vi "TAT_LABVIEW_TO_PLC_St2.vi"(7 "Enum":enum16{"Read", "Write"}(ring), 8 "error in (no error)":errorcluster, 10 "Array":bool[](array[boolean])) -> (0 "error out":errorcluster, 2 "Array 2":bool[](array[boolean]))   [LabVIEW 2017]
panel:
  # "STATION 2"
  # "SCAN OK\tM542\t\t\t2590\nSCAN NG \tM543\t\t\t2591\nSoftware on Bit\tM544\t\t\t2592\nRQST FROM TCO RESET SCAN DATA\tM545\t\t\t2593\nRepeat scan part\t\tM547\t\t2595\nPass not done station 1\t\tM548\t\t2596"
  # "34567"
  # "CONTROL PROCESS \n  LABVIEW TO PLC"
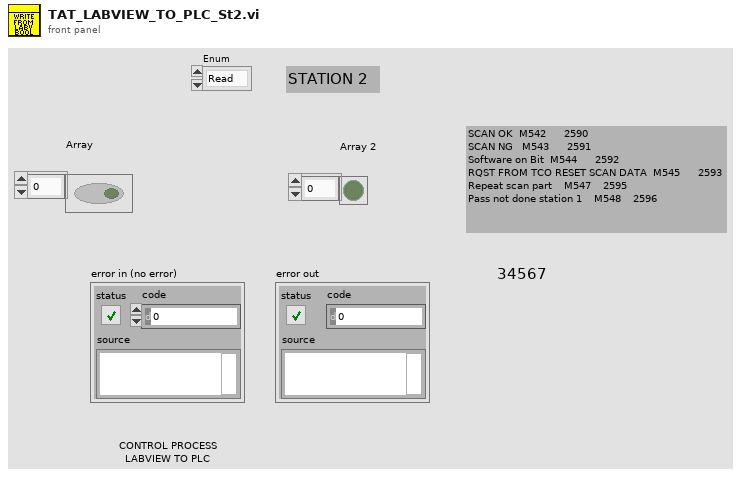
[diagram p1: front panel]
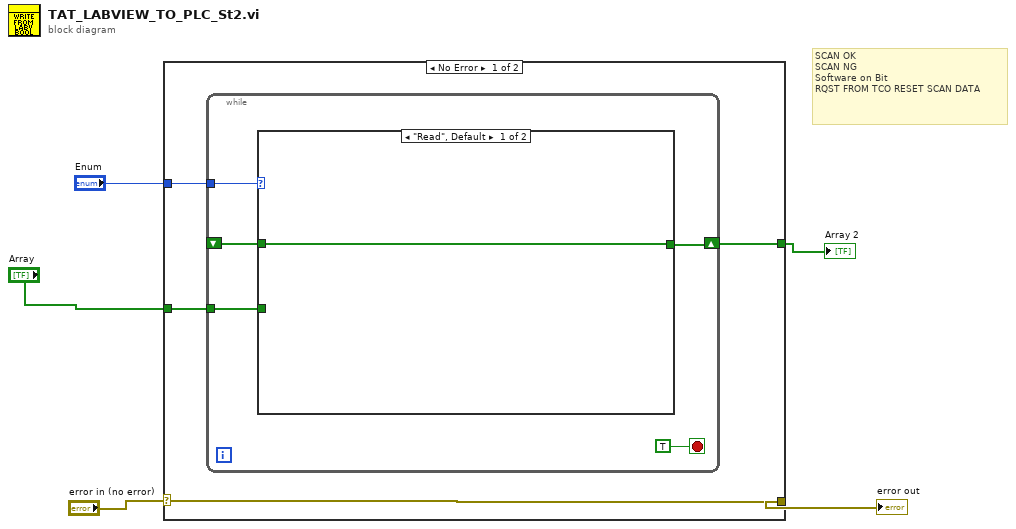
[diagram p0: block diagram]
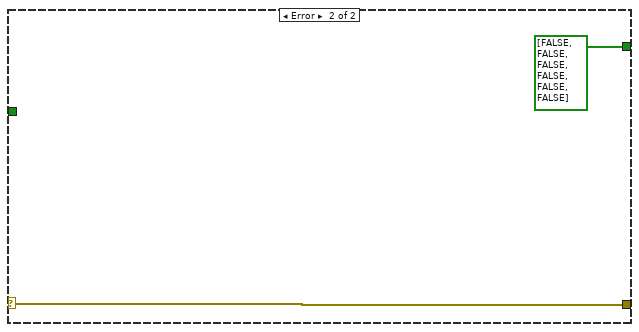
[diagram p3: hidden frame]
diagram:
  # "SCAN OK\nSCAN NG \nSoftware on Bit\nRQST FROM TCO RESET SCAN DATA"
  n1 = case shown="No Error" "error in (no error)" {
    selector: "error in (no error)" -> [w6 w18]
    tunnel: [w6 w18] -> w5
    tunnel: "Enum" -> [w9 _]
    tunnel: "Array" -> [w8 _]
    tunnel: [w7 bool[] [FALSE, FALSE, FALSE, FALSE, FALSE, FALSE]] -> w1
    frame No Error {
      n2 = while {
        tunnel: w9 -> [w13]
        shift-right: [w10] -> w7
        shift-left: _ -> [w11]
        tunnel: w8 -> [w12]
        stop <- TRUE stop-if-true
        n3 = case shown="\"Read\", Default" w13 {
          tunnel: w12 -> [_ w16]
          tunnel: [w15 w16] -> w10
          tunnel: w11 -> [w15 _]
          frame "Read", Default {
          }
          frame "Write" {
          }
        }
      }
    }
    frame Error {
    }
  }
  "error out" <- w5
  "Array 2" <- w1
